vi "Configure Sweep CCDF.vi"(6 "Sweep Cycles (125)":dbl=125.0, 7 "Enable Gated CCDF (F: Disable)":bool, 8 "error in (no error)":errorcluster, 9 "Offset Time (0 s)":dbl, 10 "Time Gate Length (0.0001 s)":dbl=0.0001, 11 "VISA resource name":refnum<visa-resource-name>) -> (0 "error out":errorcluster, 3 "VISA resource name out":refnum<visa-resource-name>)   [LabVIEW 2014, in "Agilent U2000 Series.lvlib"]
doc: "Configures the settings of Complementary Cumulative Distribution Function (CCDF) measurements for sweep mode.\n\nNote: \nThis VI is not applicable for U2040 X-Series."
uses:
  Agilent U2000 Series.lvlib
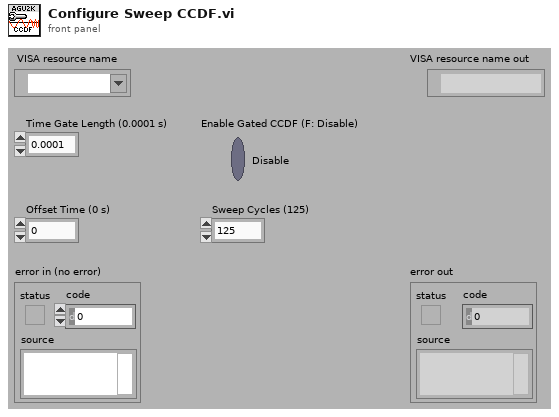
[diagram p1: front panel]
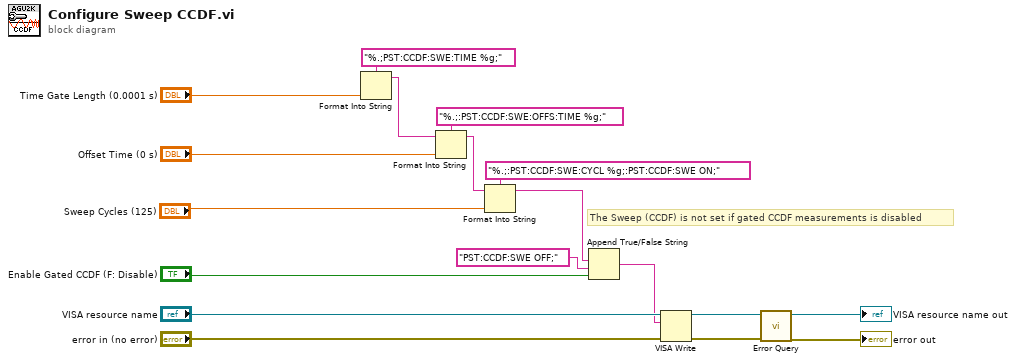
[diagram p0: block diagram]
diagram:
  # "The Sweep (CCDF) is not set if gated CCDF measurements is disabled"
  n1 = Format Into String(format string="%.;PST:CCDF:SWE:TIME %g;", "Time Gate Length (0.0001 s)") -> (resulting string=w16:string)  [unwired: 2 in, 1 out]
  n2 = Format Into String(format string="%.;:PST:CCDF:SWE:OFFS:TIME %g;", initial string=w16, "Offset Time (0 s)") -> (resulting string=w4:string)  [unwired: 1 in, 1 out]
  n3 = Format Into String(format string="%.;:PST:CCDF:SWE:CYCL %g;:PST:CCDF:SWE ON;", initial string=w4, "Sweep Cycles (125)") -> (resulting string=w3:string)  [unwired: 1 in, 1 out]
  n4 = Append True/False String(1:"Enable Gated CCDF (F: Disable)", 2:"PST:CCDF:SWE OFF;", 3:w3) -> (0:w2:string)  [unwired: 1 out]
  n5 = VISA Write(VISA resource name="VISA resource name", write buffer=w2, error in (no error)="error in (no error)") -> (VISA resource name out=w8:refnum<visa-resource-name>, error out=w7:errorcluster)  [unwired: 1 out]
  n6 = call "Error Query.vi"("error in (no error)"=w7, "VISA resource name"=w8) -> ("error out"=→"error out":errorcluster, "VISA resource name out"=→"VISA resource name out":refnum<visa-resource-name>)  [unwired: 8 out]
